vi "Update pixel info to GFG_before loading all LineScan settings.vi"(8 "error in (no error)":errorcluster, 11 "All LineScan Settings IN":T1[](array[typedef])) -> (0 "error out":errorcluster)   [LabVIEW 2012]
doc: "SciScan 1.2 160622"
uses:
  MacroGUI Module/Custom Controls and Typedefs/GFG Variable for IO.ctl
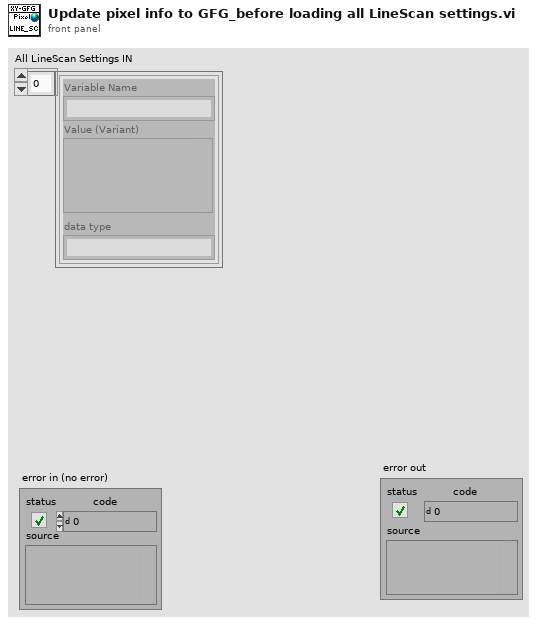
[diagram p1: front panel]
types:
  T1 = typedef "GFG Variable for IO.ctl" = cluster{"Variable Name":string, "Value (Variant)":variant, "data type":string}
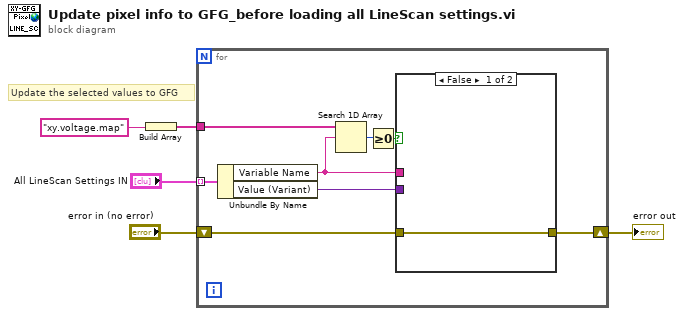
[diagram p0: block diagram]
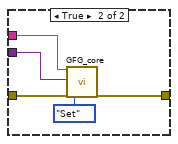
[diagram p2: hidden frame]
diagram:
  # "Update the selected values to GFG"
  n1 = Build Array("xy.voltage.map" ("Variable Name")) -> (w3:string[])
  n2 = for {
    tunnel: "All LineScan Settings IN" -> [w10] mode=indexing
    tunnel: w3 -> [w13]
    shift-right: [w6] -> w1
    shift-left: "error in (no error)" -> [w7]
    n3 = Unbundle By Name(w10) -> ("Variable Name"=w9:string, "Value (Variant)"=w8:variant)
    n4 = Search 1D Array(1D array=w13, element=w9) -> (index of element=w12:i32)  [unwired: 1 in]
    n5 = Greater Or Equal To 0?(x=w12) -> (x >= 0?=w11:bool)
    n6 = case shown="False" w11 {
      tunnel: w9 -> [_ w17]
      tunnel: w8 -> [_ w18]
      tunnel: w7 -> [w14 w16]
      tunnel: [w14 w15] -> w6
      frame False {
      }
      frame True {
        n7 = call "GFG_core.vi"("Variable Name in"=w17, "Variant in"=w18, "error in (no error)"=w16, "Action"=enum16{"Init", "Set", "Get", "Clear"}."Set") -> ("error out"=w15:errorcluster)  [unwired: 9 in, 6 out]
      }
    }
  }
  "error out" <- w1
